vi "filter-prod.vi"(7 "path tag":string="prod", 11 "files found":path[](array[path])) -> (3 "only paths containing tag":path[](array[path]))   [LabVIEW 2014]
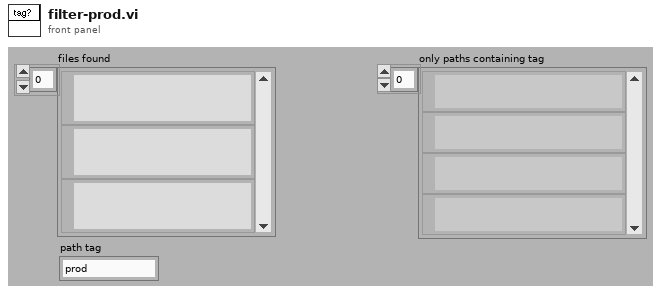
[diagram p1: front panel]
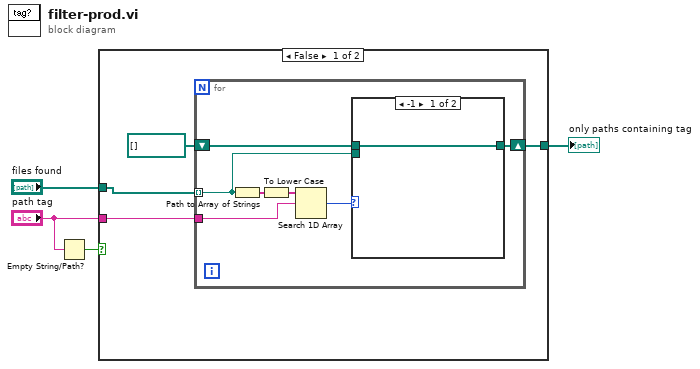
[diagram p0: block diagram]
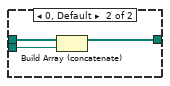
[diagram p2: hidden frame]
diagram:
  n1 = Empty String/Path?(string/path="path tag") -> (empty?=w1:bool)
  n2 = case shown="False" w1 {
    tunnel: "files found" -> [w8 w20]
    tunnel: "path tag" -> [w7 _]
    tunnel: [w5 w20] -> w3
    frame False {
      n3 = for {
        tunnel: w8 -> [w12] mode=indexing
        shift-right: [w10] -> w5
        shift-left: path[] [] -> [w11]
        tunnel: w7 -> [w14]
        n4 = Path to Array of Strings(0:w12) -> (2:w15:string[])  [unwired: 1 out]
        n5 = To Lower Case(string=w15) -> (all lower case string=w9:string[])
        n6 = Search 1D Array(1D array=w9, element=w14) -> (index of element=w13:i32)  [unwired: 1 out]
        n7 = case shown="-1" w13 {
          tunnel: w12 -> [_ w19]
          tunnel: w11 -> [w16 w18]
          tunnel: [w16 w17] -> w10
          frame -1 {
          }
          frame 0, Default {
            n8 = Build Array (concatenate)(w18, w19) -> (w17:path[])
          }
        }
      }
    }
    frame True {
    }
  }
  "only paths containing tag" <- w3
